vi "check_duplicate.vi"(11 "Array":string[](array[string])) -> (3 "hasDuplicate":bool)   [LabVIEW 2018]
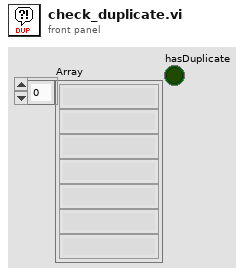
[diagram p1: front panel]
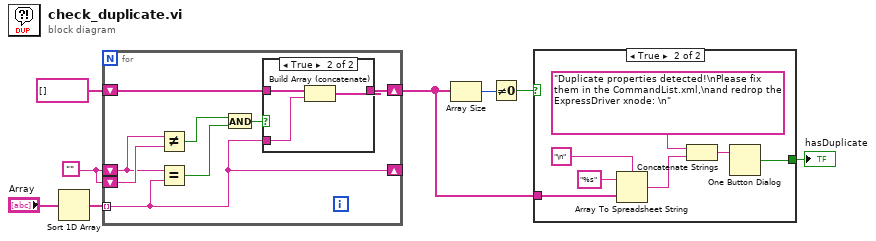
[diagram p0: block diagram]
diagram:
  w1 = ""
  n1 = Sort 1D Array(array="Array") -> (sorted array=w8:string[])
  n2 = for {
    tunnel: w8 -> [w16] mode=indexing
    shift-right: [w16] -> _
    shift-left: w1 -> [w13]
    shift-right: [w14] -> w3
    shift-left: string[] [] -> [w15]
    shift-left: w1 -> [w9]
    n3 = Not Equal?(x=w9, y=w13) -> (x != y?=w10:bool)
    n4 = Equal?(x=w9, y=w16) -> (x = y?=w11:bool)
    n5 = And(x=w10, y=w11) -> (x .and. y?=w12:bool)
    n6 = case shown="True" w12 {
      tunnel: w16 -> [_ w18]
      tunnel: [w17 w20] -> w14
      tunnel: w15 -> [w17 w19]
      frame False {
      }
      frame True {
        n7 = Build Array (concatenate)(w19, w18) -> (w20:string[])
      }
    }
  }
  n8 = Array Size(array=w3) -> (size(s)=w5:i32)
  n9 = Not Equal To 0?(x=w5) -> (x != 0?=w4:bool)
  n10 = case shown="True" w4 {
    selector: w4 -> [w21 _]
    tunnel: w3 -> [_ w28]
    tunnel: [w21 w22] -> w2
    frame False {
    }
    frame True {
      n11 = Array To Spreadsheet String(delimiter (Tab)="\n", array=w28, 3:"%s") -> (spreadsheet string=w23:string)
      n12 = Concatenate Strings("Duplicate properties detected!\nPlease fix them in the CommandList.xml,\nand redrop the ExpressDriver xnode: \n" ("string"), w23) -> (w25:string)
      n13 = One Button Dialog(message=w25) -> (true=w22:bool)  [unwired: 1 in]
    }
  }
  "hasDuplicate" <- w2
